vi "PH_DIM.Event Creator.vi"(0 "Trendnotifier Services":T1[](array[typedef]), 1 "Trendmessage Services":T1[](array[typedef]), 2 "Status Services":T1[](array[typedef]), 3 "condition Services":T1[](array[typedef]), 4 "SM State Services":T1[](array[typedef]), 5 "Data Services":T1[](array[typedef])) -> (17 "DIM Service Events":T2[](array[typedef]))   [LabVIEW 2014, in "PH_Common.lvlib"]
doc: "This VI is forseen for eased declaration of DIM Service Events. The events are of \"trendmsg\" type and; DIM services with \"Service Names\" are set to the Proc Cases at \"Service Selectors\","
uses:
  PH_Common.lvlib
  CS_Core/BaseProcess/BaseProcess.event definition.ctl
  CS_Core/CAEObj/CAEObj.event definition.ctl
  CS_Core/BaseProcess/BaseProcess.descriptor string definition.ctl
  PH_DIM.Event Declarer.ctl
  CS_Core/CAEObj/CAEObj.lvlib
  CS_Core/BaseProcess/BaseProcess.lvlib
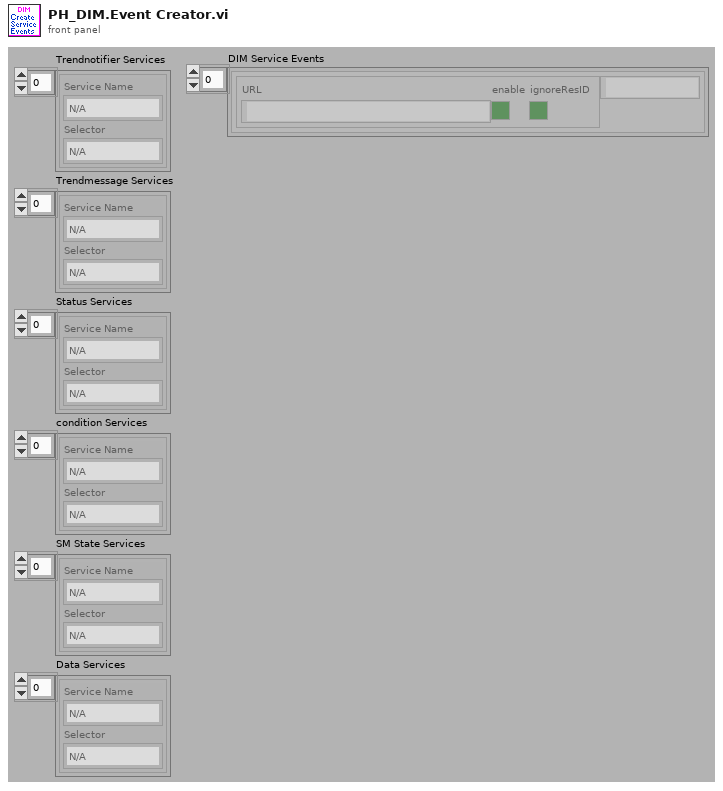
[diagram p1: front panel]
types:
  T1 = typedef "PH_Common.lvlib/PH_DIM.Event Declarer.ctl" = cluster{"Service Name":string, "Selector":string}
  T2 = typedef "BaseProcess.lvlib/BaseProcess.event definition.ctl" = cluster{"CAEEvtDef":T3, "Data Descriptor":T4}
  T3 = typedef "CAEObj.lvlib/CAEObj.event definition.ctl" = cluster{"URL":string, "enable":bool, "ignoreResID":bool}
  T4 = typedef "BaseProcess.lvlib/BaseProcess.descriptor string definition.ctl" = string
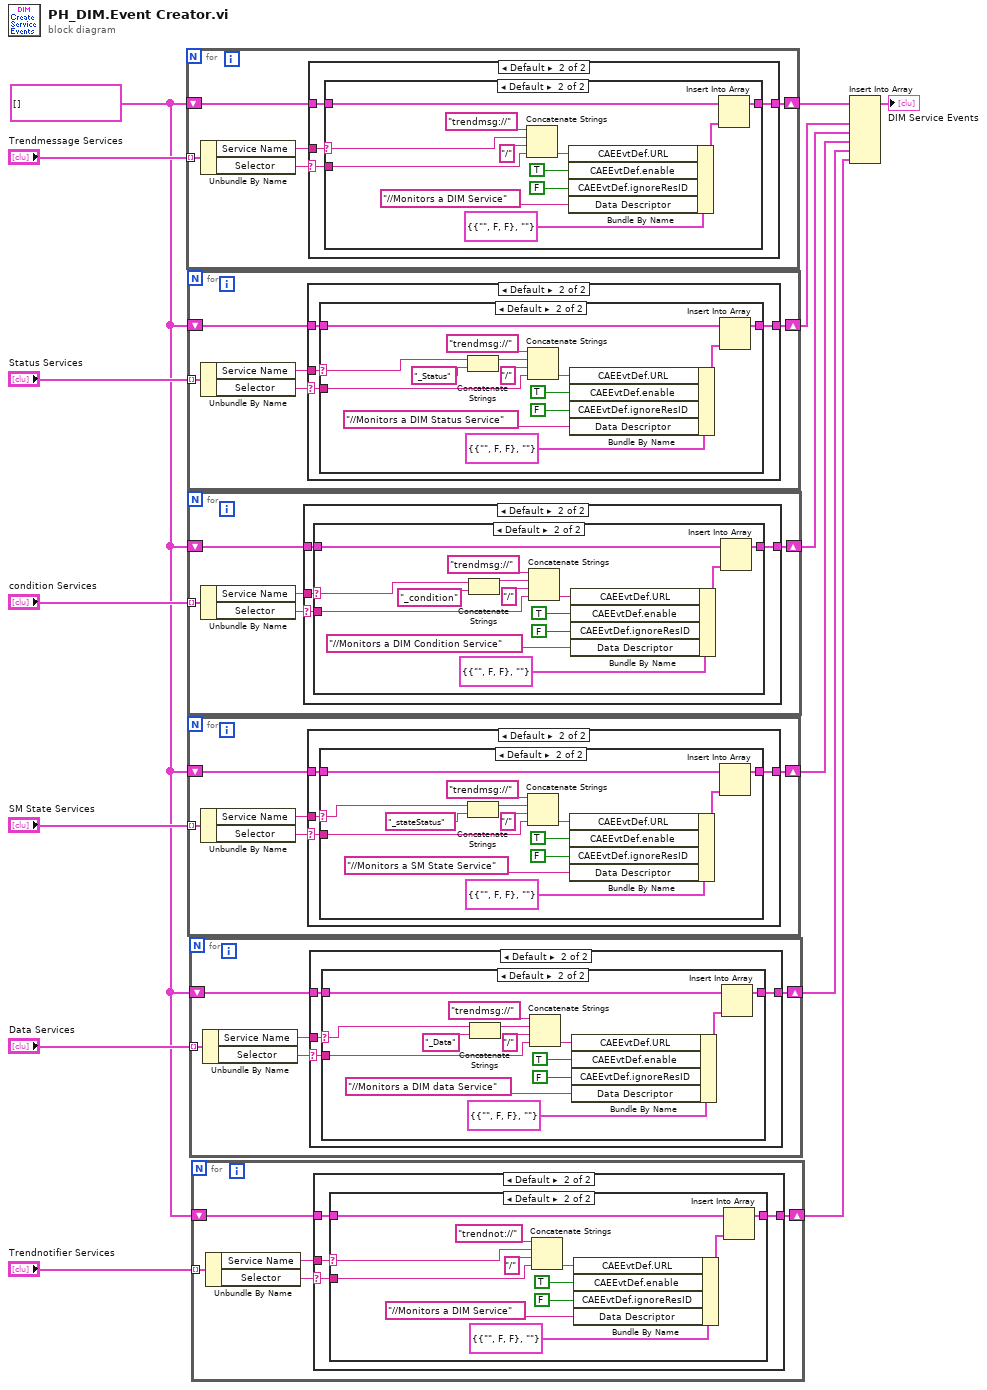
[diagram p0: block diagram]
diagram:
  w3 = T2[] [] ("new events")
  n1 = for {
    shift-right: [w19] -> w14
    shift-left: w3 -> [w18]
    tunnel: "Trendmessage Services" -> [w15] mode=indexing
    n2 = Unbundle By Name(w15) -> ("Service Name"=w16:string, "Selector"=w17:string)
    n3 = case shown="Default" w17 {
      selector: w17 -> [_ w21]
      tunnel: [w20 w24] -> w19
      tunnel: w18 -> [w20 w23]
      tunnel: w16 -> [_ w22]
      frame "N/A" {
      }
      frame Default {
        n4 = case shown="Default" w22 {
          selector: w22 -> [_ w27]
          tunnel: [w25 w37] -> w24
          tunnel: w21 -> [_ w36]
          tunnel: w23 -> [w25 w31]
          frame "N/A" {
          }
          frame Default {
            n5 = Concatenate Strings("trendmsg://" ("regular expression"), w27, "/" ("regular expression"), w36) -> (w35:string)
            n6 = Bundle By Name(cluster=T2 {"CAEEvtDef"={"URL"="", "enable"=FALSE, "ignoreResID"=FALSE}, "Data Descriptor"=""} ("Trigger"), "CAEEvtDef.URL"=w35, "CAEEvtDef.enable"=TRUE, "CAEEvtDef.ignoreResID"=FALSE, "Data Descriptor"=T4 "//Monitors a DIM Service") -> (w29:T2)
            n7 = Insert Into Array(array=w31, new element=w29) -> (w37:T2[])  [unwired: 1 in]
          }
        }
      }
    }
  }
  n8 = for {
    shift-right: [w42] -> w12
    shift-left: w3 -> [w41]
    tunnel: "Status Services" -> [w38] mode=indexing
    n9 = Unbundle By Name(w38) -> ("Service Name"=w40:string, "Selector"=w39:string)
    n10 = case shown="Default" w39 {
      selector: w39 -> [_ w44]
      tunnel: [w43 w47] -> w42
      tunnel: w41 -> [w43 w46]
      tunnel: w40 -> [_ w45]
      frame "N/A" {
      }
      frame Default {
        n11 = case shown="Default" w45 {
          selector: w45 -> [_ w50]
          tunnel: [w48 w62] -> w47
          tunnel: w44 -> [_ w61]
          tunnel: w46 -> [w48 w56]
          frame "N/A" {
          }
          frame Default {
            n12 = Concatenate Strings(w50, "_Status" ("string")) -> (w51:string)
            n13 = Concatenate Strings("trendmsg://" ("regular expression"), w51, "/" ("regular expression"), w61) -> (w60:string)
            n14 = Bundle By Name(cluster=T2 {"CAEEvtDef"={"URL"="", "enable"=FALSE, "ignoreResID"=FALSE}, "Data Descriptor"=""} ("Trigger"), "CAEEvtDef.URL"=w60, "CAEEvtDef.enable"=TRUE, "CAEEvtDef.ignoreResID"=FALSE, "Data Descriptor"=T4 "//Monitors a DIM Status Service") -> (w54:T2)
            n15 = Insert Into Array(array=w56, new element=w54) -> (w62:T2[])  [unwired: 1 in]
          }
        }
      }
    }
  }
  n16 = for {
    shift-right: [w67] -> w11
    shift-left: w3 -> [w66]
    tunnel: "condition Services" -> [w63] mode=indexing
    n17 = Unbundle By Name(w63) -> ("Service Name"=w65:string, "Selector"=w64:string)
    n18 = case shown="Default" w64 {
      selector: w64 -> [_ w69]
      tunnel: [w68 w72] -> w67
      tunnel: w66 -> [w68 w71]
      tunnel: w65 -> [_ w70]
      frame "N/A" {
      }
      frame Default {
        n19 = case shown="Default" w70 {
          selector: w70 -> [_ w74]
          tunnel: [w73 w87] -> w72
          tunnel: w69 -> [_ w86]
          tunnel: w71 -> [w73 w81]
          frame "N/A" {
          }
          frame Default {
            n20 = Concatenate Strings(w74, "_condition" ("string")) -> (w75:string)
            n21 = Concatenate Strings("trendmsg://" ("regular expression"), w75, "/" ("regular expression"), w86) -> (w85:string)
            n22 = Bundle By Name(cluster=T2 {"CAEEvtDef"={"URL"="", "enable"=FALSE, "ignoreResID"=FALSE}, "Data Descriptor"=""} ("Trigger"), "CAEEvtDef.URL"=w85, "CAEEvtDef.enable"=TRUE, "CAEEvtDef.ignoreResID"=FALSE, "Data Descriptor"=T4 "//Monitors a DIM Condition Service") -> (w79:T2)
            n23 = Insert Into Array(array=w81, new element=w79) -> (w87:T2[])  [unwired: 1 in]
          }
        }
      }
    }
  }
  n24 = for {
    shift-right: [w92] -> w6
    shift-left: w3 -> [w91]
    tunnel: "SM State Services" -> [w88] mode=indexing
    n25 = Unbundle By Name(w88) -> ("Service Name"=w90:string, "Selector"=w89:string)
    n26 = case shown="Default" w89 {
      selector: w89 -> [_ w94]
      tunnel: [w93 w97] -> w92
      tunnel: w91 -> [w93 w96]
      tunnel: w90 -> [_ w95]
      frame "N/A" {
      }
      frame Default {
        n27 = case shown="Default" w95 {
          selector: w95 -> [_ w100]
          tunnel: [w98 w112] -> w97
          tunnel: w94 -> [_ w111]
          tunnel: w96 -> [w98 w106]
          frame "N/A" {
          }
          frame Default {
            n28 = Concatenate Strings(w100, "_stateStatus" ("string")) -> (w101:string)
            n29 = Concatenate Strings("trendmsg://" ("regular expression"), w101, "/" ("regular expression"), w111) -> (w110:string)
            n30 = Bundle By Name(cluster=T2 {"CAEEvtDef"={"URL"="", "enable"=FALSE, "ignoreResID"=FALSE}, "Data Descriptor"=""} ("Trigger"), "CAEEvtDef.URL"=w110, "CAEEvtDef.enable"=TRUE, "CAEEvtDef.ignoreResID"=FALSE, "Data Descriptor"=T4 "//Monitors a SM State Service") -> (w104:T2)
            n31 = Insert Into Array(array=w106, new element=w104) -> (w112:T2[])  [unwired: 1 in]
          }
        }
      }
    }
  }
  n32 = for {
    shift-right: [w117] -> w4
    shift-left: w3 -> [w116]
    tunnel: "Data Services" -> [w113] mode=indexing
    n33 = Unbundle By Name(w113) -> ("Service Name"=w115:string, "Selector"=w114:string)
    n34 = case shown="Default" w114 {
      selector: w114 -> [_ w119]
      tunnel: [w118 w122] -> w117
      tunnel: w116 -> [w118 w121]
      tunnel: w115 -> [_ w120]
      frame "N/A" {
      }
      frame Default {
        n35 = case shown="Default" w120 {
          selector: w120 -> [_ w125]
          tunnel: [w123 w137] -> w122
          tunnel: w119 -> [_ w136]
          tunnel: w121 -> [w123 w131]
          frame "N/A" {
          }
          frame Default {
            n36 = Concatenate Strings(w125, "_Data" ("string")) -> (w126:string)
            n37 = Concatenate Strings("trendmsg://" ("regular expression"), w126, "/" ("regular expression"), w136) -> (w135:string)
            n38 = Bundle By Name(cluster=T2 {"CAEEvtDef"={"URL"="", "enable"=FALSE, "ignoreResID"=FALSE}, "Data Descriptor"=""} ("Trigger"), "CAEEvtDef.URL"=w135, "CAEEvtDef.enable"=TRUE, "CAEEvtDef.ignoreResID"=FALSE, "Data Descriptor"=T4 "//Monitors a DIM data Service") -> (w129:T2)
            n39 = Insert Into Array(array=w131, new element=w129) -> (w137:T2[])  [unwired: 1 in]
          }
        }
      }
    }
  }
  n40 = for {
    shift-right: [w142] -> w1
    shift-left: w3 -> [w141]
    tunnel: "Trendnotifier Services" -> [w138] mode=indexing
    n41 = Unbundle By Name(w138) -> ("Service Name"=w139:string, "Selector"=w140:string)
    n42 = case shown="Default" w140 {
      selector: w140 -> [_ w144]
      tunnel: [w143 w147] -> w142
      tunnel: w141 -> [w143 w146]
      tunnel: w139 -> [_ w145]
      frame "N/A" {
      }
      frame Default {
        n43 = case shown="Default" w145 {
          selector: w145 -> [_ w150]
          tunnel: [w148 w160] -> w147
          tunnel: w144 -> [_ w159]
          tunnel: w146 -> [w148 w154]
          frame "N/A" {
          }
          frame Default {
            n44 = Concatenate Strings("trendnot://" ("regular expression"), w150, "/" ("regular expression"), w159) -> (w158:string)
            n45 = Bundle By Name(cluster=T2 {"CAEEvtDef"={"URL"="", "enable"=FALSE, "ignoreResID"=FALSE}, "Data Descriptor"=""} ("Trigger"), "CAEEvtDef.URL"=w158, "CAEEvtDef.enable"=TRUE, "CAEEvtDef.ignoreResID"=FALSE, "Data Descriptor"=T4 "//Monitors a DIM Service") -> (w152:T2)
            n46 = Insert Into Array(array=w154, new element=w152) -> (w160:T2[])  [unwired: 1 in]
          }
        }
      }
    }
  }
  n47 = Insert Into Array(array=w14, new element #1=w12, new element #2=w11, new element #3=w6, new element #4=w4, new element #5=w1) -> (→"DIM Service Events":T2[])  [unwired: 1 in]
